vi "AE_trigger_wPlot.vi"() -> ()   [LabVIEW 2012]
uses:
  <vilib>/DAQmx/read.llb/DAQmx Read (Analog 1D Wfm NChan NSamp).vi
  <vilib>/DAQmx/create/channels.llb/DAQmx Create Channel (AI-Voltage-Basic).vi
  <vilib>/DAQmx/configure/timing.llb/DAQmx Timing (Sample Clock).vi
  <vilib>/DAQmx/configure/trigger.llb/DAQmx Reference Trigger (Analog Edge).vi
  <vilib>/DAQmx/miscellaneous.llb/DAQmx Fill In Error Info.vi
panel:
  out "Wavelets":waveform(dbl)[](graph)
  in  "Trigger (V)":dbl=0.01 min=0.0 max=10.0 step=0.001 format="%0.3f"
  in  "Physical Channel":tag="Dev1/ai7"
  in  "Gain":u16(ring)=1 items=["20 dB", "40 dB", "60 dB"]
  out "Events":i32
  in  "Sample Window (us)":i32=500 min=0 max=1000
  in  "stop":bool
  in  "Test Name":string="test"
  in  "Storage Directory":path=path "C:/Users/User/Desktop/Users_2013-2014/Michael Rossol"
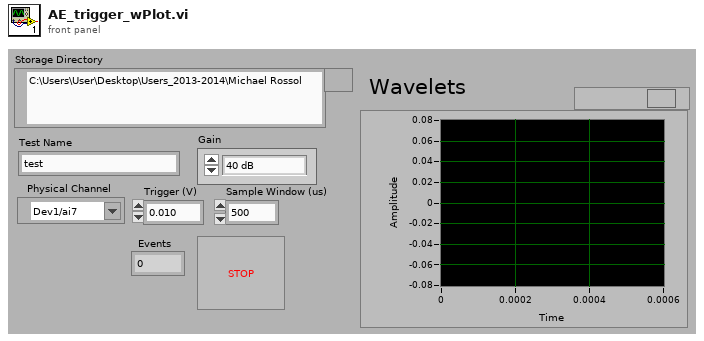
[diagram p1: front panel]
types:
  T1 = enum16{"open", "open or create", "create or replace", "create", "open (read only)"}
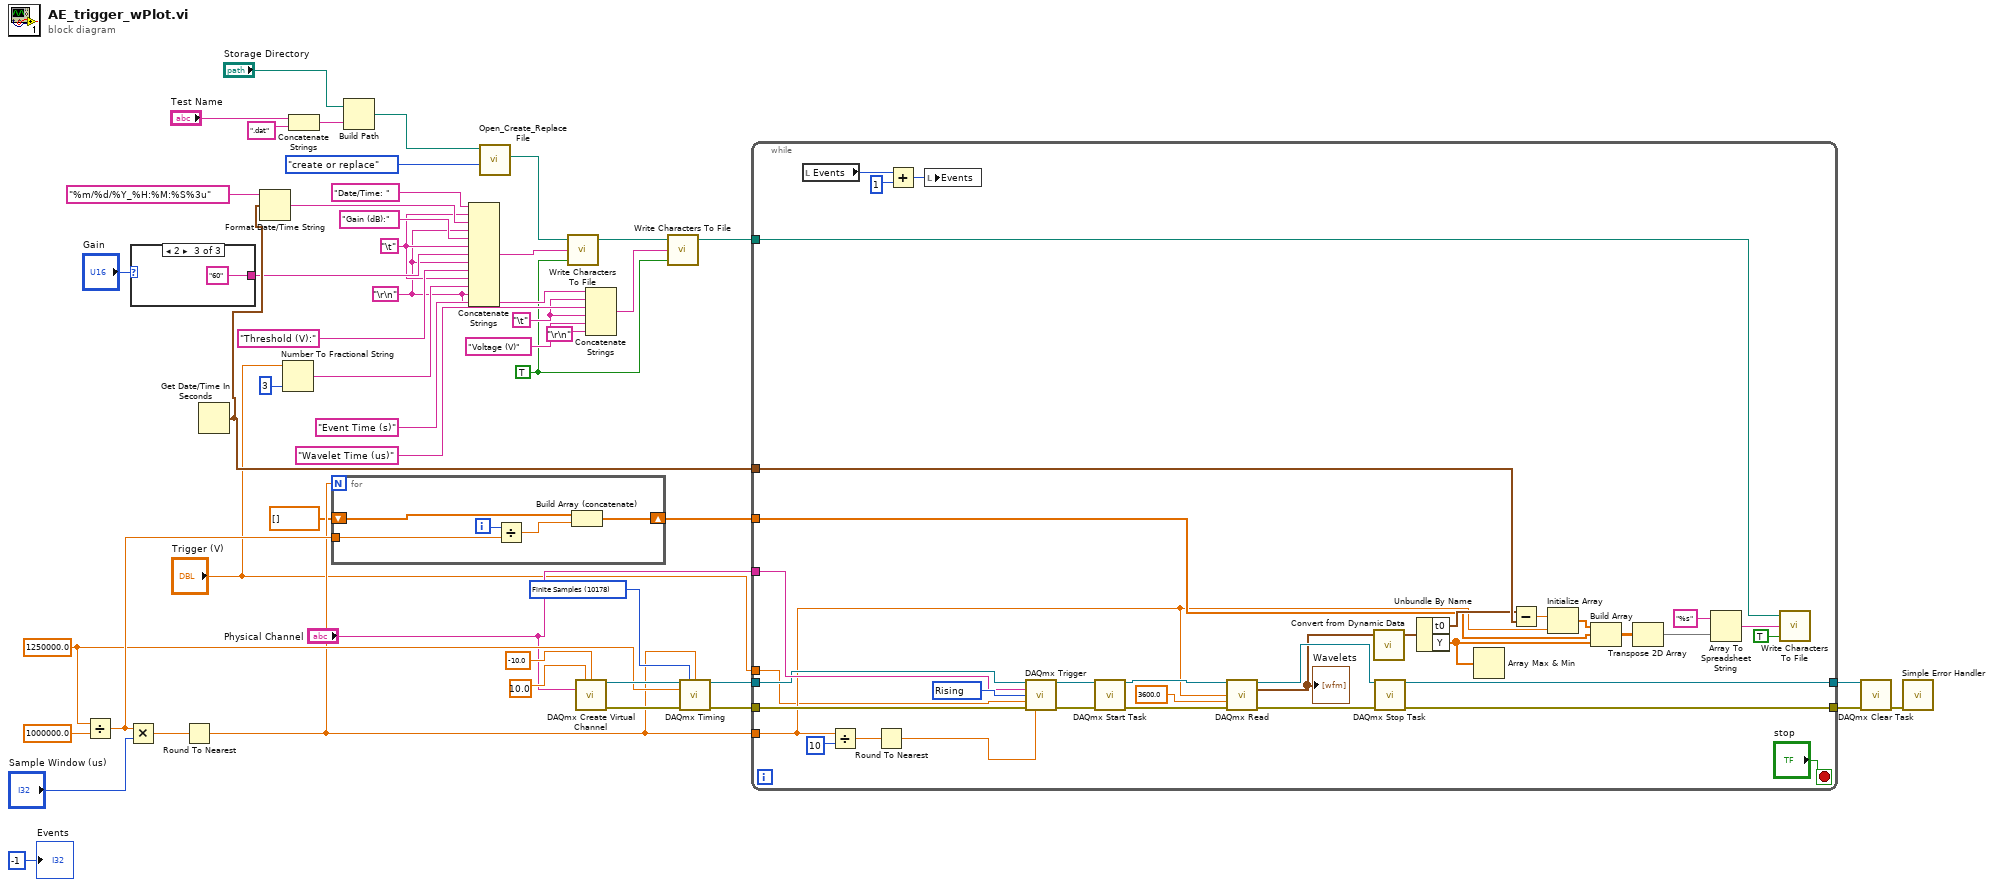
[diagram p0: block diagram]
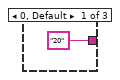
[diagram p2: hidden frame]
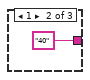
[diagram p3: hidden frame]
diagram:
  w18 = 10178 items=["Finite Samples"=10178, "Continuous Samples"=10123] ("sample mode")
  w32 = "\t"
  w17 = 1250000.0 ("x")
  w5 = "\t"
  w1 = "\r\n"
  w29 = TRUE ("append to file? (new file:F)")
  n1 = Divide(x=w17, y=1000000.0) -> (x/y=w35:dbl)
  n2 = Multiply(x=w35, y="Sample Window (us)") -> (x*y=w11:dbl)
  n3 = case shown="2" "Gain" {
    tunnel: ["20" ("string") "40" ("string") "60" ("string")] -> w23
    frame 0, Default {
    }
    frame 1 {
    }
    frame 2 {
    }
  }
  n4 = Round To Nearest(number=w11) -> (nearest integer value=w10:dbl)
  n5 = Get Date/Time In Seconds() -> (seconds since 1Jan1904=w36:timestamp)
  n6 = Format Date/Time String(time format string (%c)="%m/%d/%Y_%H:%M:%S%3u", seconds (now)=w36) -> (date/time string=w40:string)  [unwired: 1 in]
  n7 = Number To Fractional String(number="Trigger (V)", precision (6)=i16 3) -> (F-format string=w2:string)  [unwired: 2 in]
  n8 = Concatenate Strings("Test Name", ".dat" ("string")) -> (w43:string)
  n9 = for {
    N: w10 -> [_]
    shift-right: [w57] -> w9
    shift-left: dbl[] [] -> [w58]
    tunnel: w35 -> [w54]
    i -> [w56]
    n10 = Divide(x=w56, y=w54) -> (x/y=w55:dbl)
    n11 = Build Array (concatenate)(w58, w55) -> (w57:dbl[])
  }
  n12 = Build Path(base path="Storage Directory", name or relative path=w43) -> (appended path=w41:path)
  n13 = Concatenate Strings("Date/Time: ", w5, w40, w1, "Gain (dB):" ("string"), w5, w23, w1, "Threshold (V):" ("string"), w5, w2, w1, w1) -> (w50:string)
  n14 = call <vilib>:"Open_Create_Replace File.vi"("function (open:0)"=T1."create or replace", "file path"=w41) -> ("new file path"=w46:path)  [unwired: 6 in, 3 out]
  n15 = call <vilib>:"Write Characters To File.vi"("append to file? (new file:F)"=w29, "character string"=w50, "file path (dialog if empty)"=w46) -> ("new file path (Not A Path if cancelled)"=w27:path)  [unwired: 2 in]
  n16 = call-poly <vilib>:"DAQmx Create Virtual Channel.vi"("maximum value"=10.0, "minimum value"=-10.0, "physical channels"="Physical Channel") -> ("task out"=w20:refnum<k21>, "error out"=w19:errorcluster)  [unwired: 11 in]
  n17 = Concatenate Strings("Event Time (s)" ("string"), w32, "Wavelet Time (us)" ("string"), w32, "Voltage (V)" ("string"), "\r\n") -> (w28:string)
  n18 = call <vilib>:"Write Characters To File.vi"("append to file? (new file:F)"=w29, "character string"=w28, "file path (dialog if empty)"=w27) -> ("new file path (Not A Path if cancelled)"=w26:path)  [unwired: 2 in]
  n19 = call-poly <vilib>:"DAQmx Timing.vi"("task/channels in"=w20, "sample mode"=w18, "samples per channel"=w10, "rate"=w17, "error in"=w19) -> ("task out"=w16:refnum<k21>, "error out"=w15:errorcluster)  [unwired: 9 in]
  n20 = while {
    tunnel: w26 -> [w91]
    tunnel: w10 -> [w63]
    tunnel: w36 -> [w85]
    tunnel: w9 -> [w79]
    tunnel: w16 -> [w70]
    tunnel: w15 -> [w69]
    tunnel: [w75] -> w13
    tunnel: [w74] -> w12
    tunnel: "Physical Channel" -> [w72]
    tunnel: "Trigger (V)" -> [w59]
    stop <- "stop" stop-if-true
    w73 = 10280 items=["Rising"=10280, "Falling"=10171] ("slope")
    n21 = local read "Events"() -> (w89:i32)
    n22 = Divide(x=w63, y=u32 10 ("pretrigger samples per channel")) -> (x/y=w60:dbl)
    n23 = Round To Nearest(number=w60) -> (nearest integer value=w61:dbl)
    n24 = Add(x=w89, y=1) -> (x+y=w88:i32)
    n25 = local write "Events"(w88) -> ()
    n26 = call-poly <vilib>:"DAQmx Trigger.vi"("task/channels in"=w70, "source"=w72, "slope"=w73, "level"=w59, "error in"=w69, "pretrigger samples per channel"=w61) -> ("task out"=w68:refnum<k21>, "error out"=w65:errorcluster)  [unwired: 8 in]
    n27 = call <vilib>:"DAQmx Start Task.vi"("task/channels in"=w68, "error in"=w65) -> ("task out"=w67:refnum<k21>, "error out"=w66:errorcluster)  [unwired: 12 in]
    n28 = call-poly <vilib>:"DAQmx Read.vi"("task/channels in"=w67, "number of samples per channel"=w63, "timeout"=3600.0, "error in"=w66) -> ("task out"=w76:refnum<k21>, "data"=w62:waveform(dbl)[], "error out"=w77:errorcluster)  [unwired: 9 in]
    "Wavelets" <- w62
    n29 = call "Convert from Dynamic Data"("Dynamic Data Type"=w62) -> ("Waveform"=w86:waveform(dbl))  [unwired: 3 in]
    n30 = call <vilib>:"DAQmx Stop Task.vi"("task/channels in"=w76, "error in"=w77) -> ("task out"=w74:refnum<k21>, "error out"=w75:errorcluster)  [unwired: 12 in]
    n31 = Unbundle By Name(w86) -> ("t0"=w84:timestamp, "Y"=w71:dbl[])
    n32 = Array Max & Min(array=w71) -> ()  [unwired: 4 out]
    n33 = Subtract(x=w84, y=w85) -> (x-y=w83:dbl)
    n34 = Initialize Array(w83, w63) -> (w82:dbl[])
    n35 = Build Array(w82, w79, w71) -> (w81:dbl[][])
    n36 = Transpose 2D Array(2D array=w81) -> (transposed array=w80:dbl[][])
    n37 = Array To Spreadsheet String(array=w80, 3:"%s" ("format string")) -> (spreadsheet string=w92:string)  [unwired: 1 in]
    n38 = call <vilib>:"Write Characters To File.vi"("append to file? (new file:F)"=TRUE, "character string"=w92, "file path (dialog if empty)"=w91) -> ()  [unwired: 2 in, 1 out]
  }
  n39 = call <vilib>:"DAQmx Clear Task.vi"("task in"=w12, "error in"=w13) -> ("error out"=w14:errorcluster)  [unwired: 13 in]
  n40 = call <vilib>:"Simple Error Handler.vi"("error in (no error)"=w14) -> ()  [unwired: 4 in, 5 out]
  "Events" <- -1
